vi "Decimal_to_boolean(input).vi"(1 "conInput":i8) -> (0 "dig IO":bool[](array[boolean]))   [LabVIEW 2010]
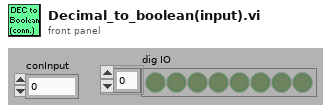
[diagram p1: front panel]
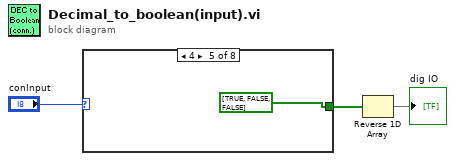
[diagram p0: block diagram]
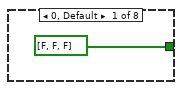
[diagram p2: hidden frame]
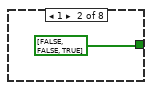
[diagram p3: hidden frame]
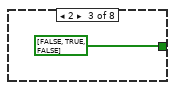
[diagram p4: hidden frame]
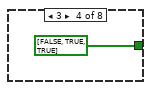
[diagram p5: hidden frame]
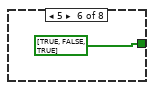
[diagram p6: hidden frame]
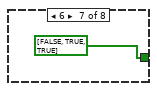
[diagram p7: hidden frame]
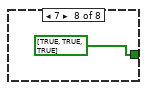
[diagram p8: hidden frame]
diagram:
  n1 = case shown="4" "conInput" {
    tunnel: [bool[] [FALSE, FALSE, FALSE] ("data") bool[] [FALSE, FALSE, TRUE] ("data") bool[] [FALSE, TRUE, FALSE] ("data") bool[] [FALSE, TRUE, TRUE] ("data") bool[] [TRUE, FALSE, FALSE] ("data") bool[] [TRUE, FALSE, TRUE] ("data") bool[] [FALSE, TRUE, TRUE] ("data") bool[] [TRUE, TRUE, TRUE] ("data")] -> w2
    frame 0, Default {
    }
    frame 1 {
    }
    frame 2 {
    }
    frame 3 {
    }
    frame 4 {
    }
    frame 5 {
    }
    frame 6 {
    }
    frame 7 {
    }
  }
  n2 = Reverse 1D Array(array=w2) -> (reversed array=→"dig IO":bool[])
